vi "FileRichInfo2StringBySecond.vi"(0 "file path (dialog if empty)":path caption="文件路径 （空时为对话框）", 1 "BeginTime(s)":dbl, 2 "EndTime(s)":dbl, 3 "总帧数":i32, 4 "文件类型":string="unknown", 5 "Language":u32) -> (8 "FileInfo":string)   [LabVIEW 2015]
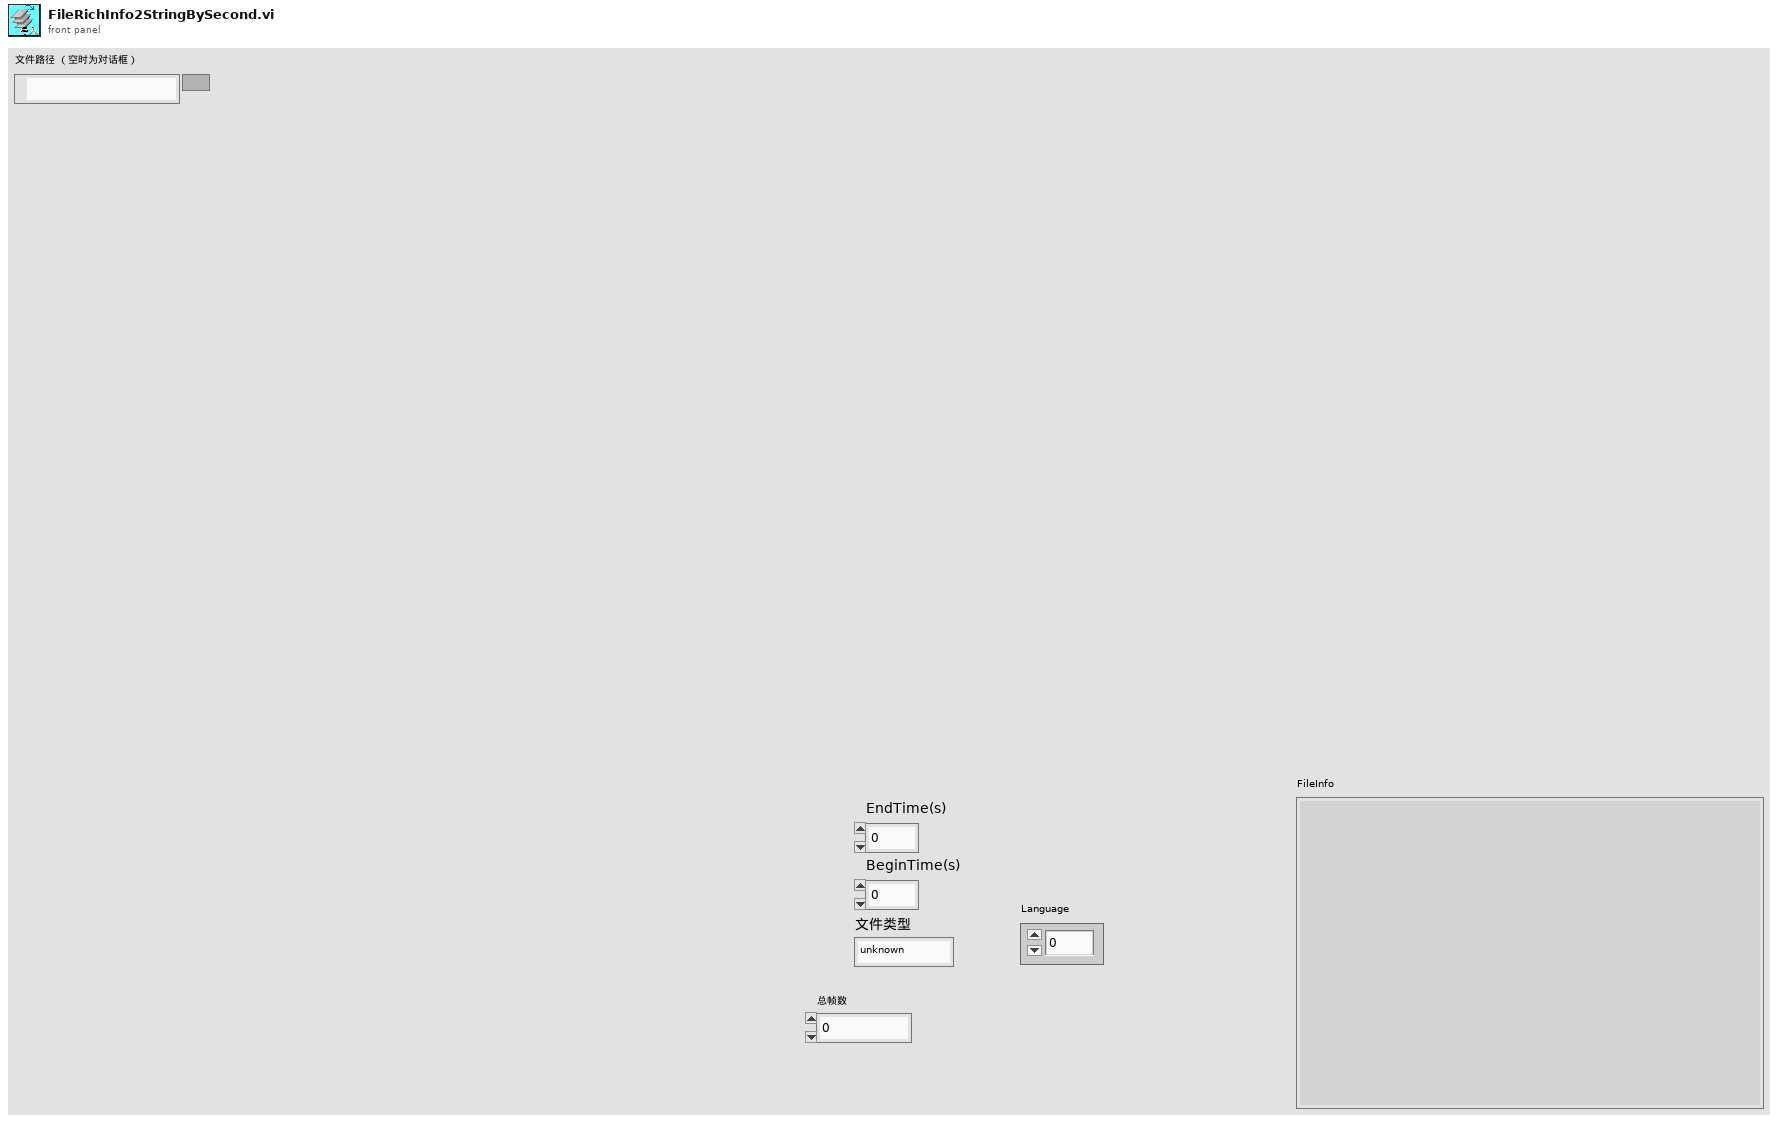
[diagram p1: front panel]
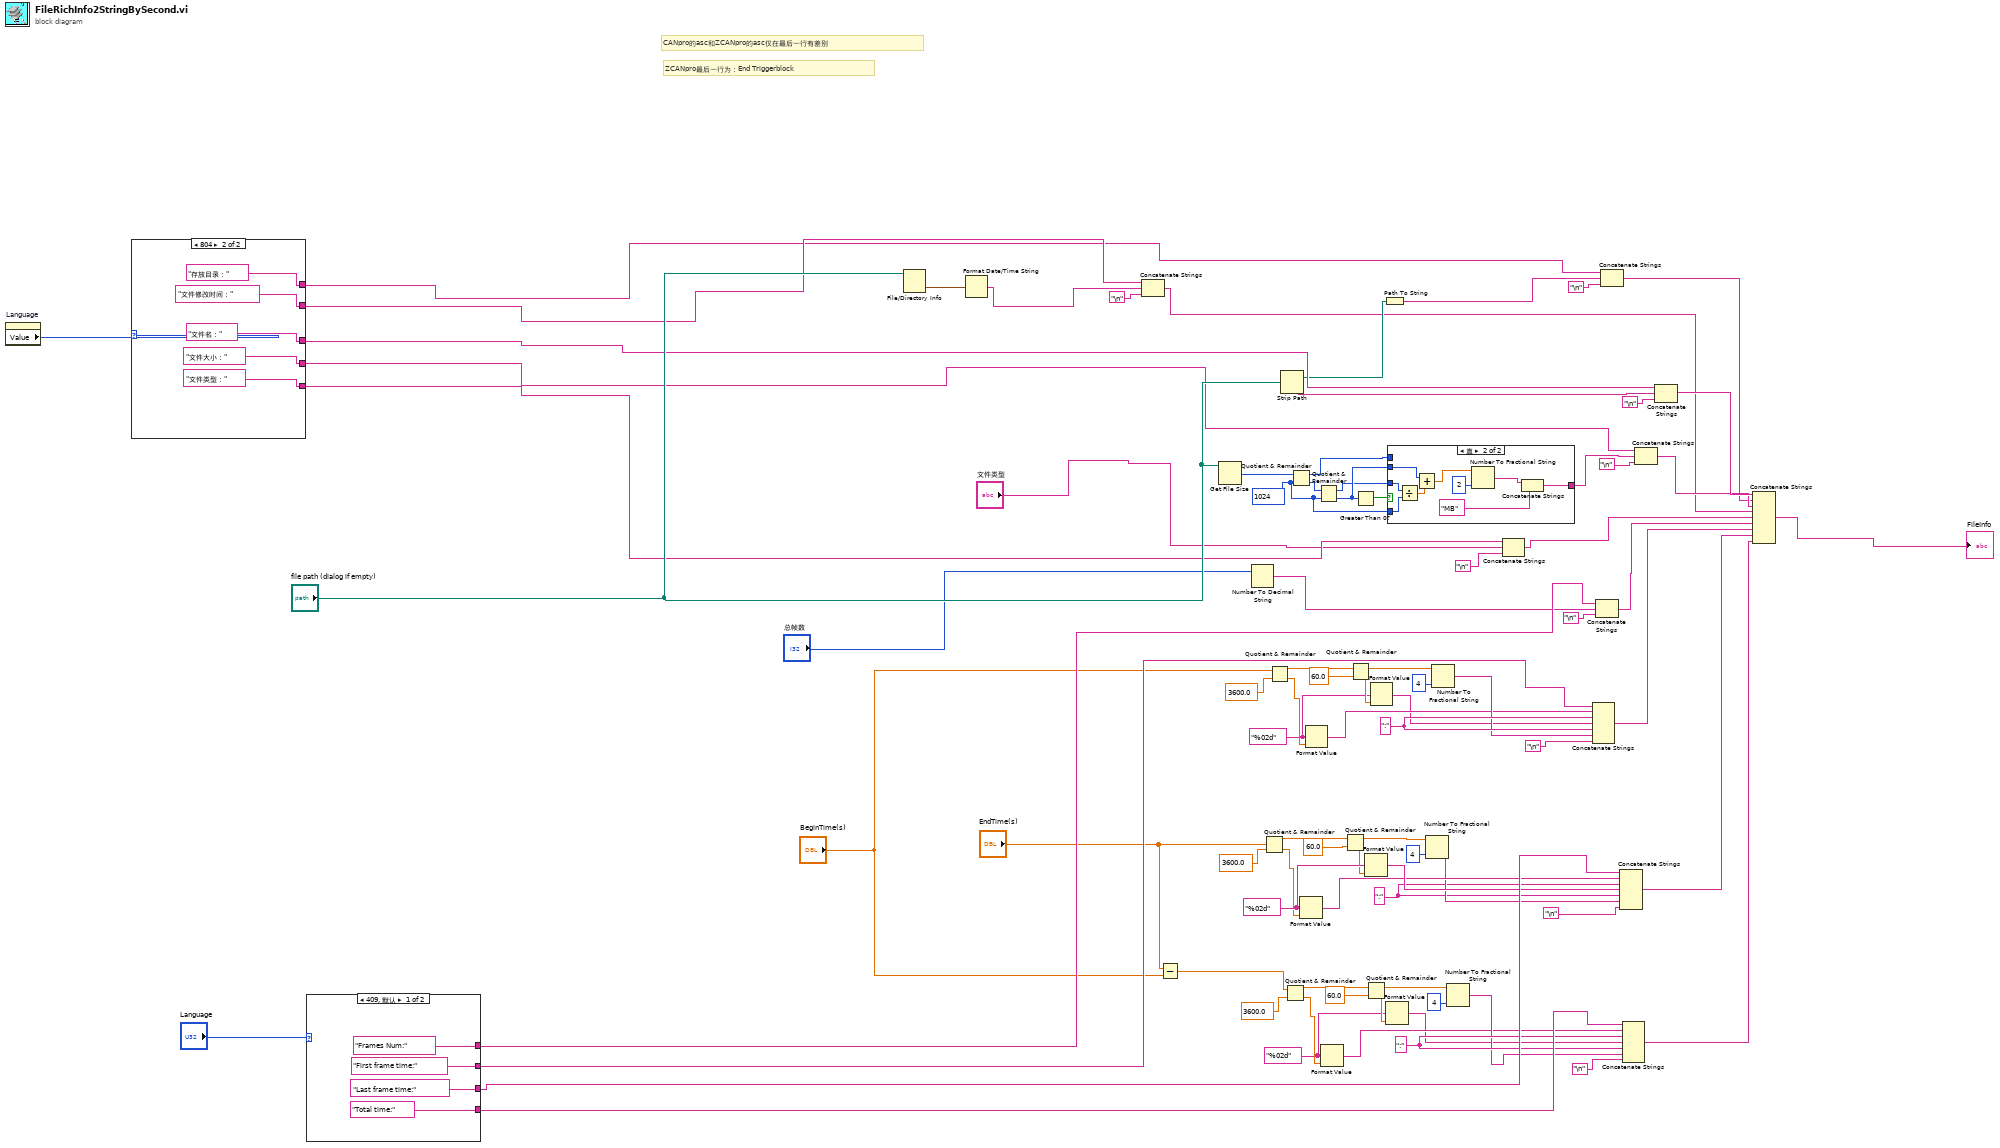
[diagram p0: block diagram]
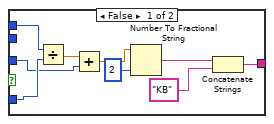
[diagram p2: hidden frame]
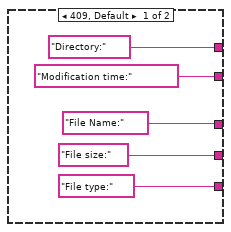
[diagram p3: hidden frame]
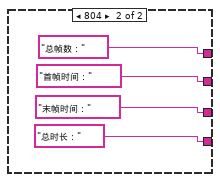
[diagram p4: hidden frame]
diagram:
  w17 = i64 1024 ("y")
  w36 = "%02d" ("格式字符串")
  w42 = ":"
  w60 = "%02d" ("格式字符串")
  w54 = ":"
  w62 = "%02d" ("格式字符串")
  w68 = ":"
  # "ZCANpro最后一行为：End Triggerblock"
  # "CANpro的asc和ZCANpro的asc仅在最后一行有差别"
  n1 = property on="Language" class="DigNum (严格)"() -> ("Value"=w83:u32)  [unwired: 2 in, 2 out]
  n2 = case shown="804" w83 {
    tunnel: ["Modification time:" "文件修改时间："] -> w82
    tunnel: ["Directory:" "存放目录："] -> w79
    tunnel: ["File Name:" "文件名："] -> w80
    tunnel: ["File size:" "文件大小："] -> w78
    tunnel: ["File type:" "文件类型："] -> w81
    frame 409, Default {
    }
    frame 804 {
    }
  }
  n3 = case shown="409, 默认" "Language" {
    tunnel: ["Total time:" "总时长："] -> w77
    tunnel: ["Last frame time:" "末帧时间："] -> w76
    tunnel: ["First frame time:" "首帧时间："] -> w75
    tunnel: ["Frames Num:" "总帧数："] -> w74
    frame 409, Default {
    }
    frame 804 {
    }
  }
  n4 = File/Directory Info(path="file path (dialog if empty)") -> (last mod=w8:timestamp)  [unwired: 1 in, 6 out]
  n5 = Format Date/Time String(seconds (now)=w8) -> (date/time string=w6:string)  [unwired: 2 in]
  n6 = Concatenate Strings(w82, w6, "\n") -> (w5:string)
  n7 = Subtract(x="EndTime(s)", y="BeginTime(s)") -> (x-y=w35:dbl)
  n8 = Get File Size(file="file path (dialog if empty)") -> (size (in bytes)=w20:i64)  [unwired: 1 in, 2 out]
  n9 = Number To Decimal String(number="总帧数") -> (decimal integer string=w23:string)  [unwired: 1 in]
  n10 = Quotient & Remainder(x="EndTime(s)", y=3600.0) -> (x-y*floor(x/y)=w50:dbl, floor(x/y)=w57:dbl)
  n11 = Quotient & Remainder(x="BeginTime(s)", y=3600.0) -> (x-y*floor(x/y)=w72:dbl, floor(x/y)=w65:dbl)
  n12 = Strip Path(path="file path (dialog if empty)") -> (stripped path=w10:path, name=w30:string)
  n13 = Quotient & Remainder(x=w35, y=3600.0) -> (x-y*floor(x/y)=w46:dbl, floor(x/y)=w39:dbl)
  n14 = Quotient & Remainder(x=w20, y=w17) -> (x-y*floor(x/y)=w13:i64, floor(x/y)=w19:i64)
  n15 = Format Value(format string=w60, value (0)=w57) -> (output string=w56:string)  [unwired: 1 in]
  n16 = Format Value(format string=w62, value (0)=w65) -> (output string=w66:string)  [unwired: 1 in]
  n17 = Quotient & Remainder(x=w19, y=w17) -> (x-y*floor(x/y)=w15:i64, floor(x/y)=w16:i64)
  n18 = Format Value(format string=w36, value (0)=w39) -> (output string=w40:string)  [unwired: 1 in]
  n19 = Quotient & Remainder(x=w50, y=60.0) -> (x-y*floor(x/y)=w52:dbl, floor(x/y)=w58:dbl)
  n20 = Quotient & Remainder(x=w72, y=60.0) -> (x-y*floor(x/y)=w70:dbl, floor(x/y)=w64:dbl)
  n21 = Greater Than 0?(x=w16) -> (x > 0?=w18:bool)
  n22 = Format Value(format string=w60, value (0)=w58) -> (output string=w59:string)  [unwired: 1 in]
  n23 = Quotient & Remainder(x=w46, y=60.0) -> (x-y*floor(x/y)=w44:dbl, floor(x/y)=w38:dbl)
  n24 = Format Value(format string=w62, value (0)=w64) -> (output string=w63:string)  [unwired: 1 in]
  n25 = Path To String(path=w10) -> (string=w11:string)
  n26 = Format Value(format string=w36, value (0)=w38) -> (output string=w37:string)  [unwired: 1 in]
  n27 = case shown="真" w18 {
    tunnel: w17 -> [w110 w120]
    tunnel: w16 -> [_ w118]
    tunnel: w15 -> [w108 w121]
    tunnel: [w113 w116] -> w14
    tunnel: w13 -> [w111 _]
    frame False {
      n28 = Divide(x=w111, y=w110) -> (x/y=w109:dbl)
      n29 = Add(x=w109, y=w108) -> (x+y=w107:dbl)
      n30 = Number To Fractional String(number=w107, precision (6)=i16 2 ("精度(6)")) -> (F-format string=w105:string)  [unwired: 2 in]
      n31 = Concatenate Strings(w105, "KB" ("字符串")) -> (w113:string)
    }
    frame True {
      n32 = Divide(x=w121, y=w120) -> (x/y=w119:dbl)
      n33 = Add(x=w118, y=w119) -> (x+y=w117:dbl)
      n34 = Number To Fractional String(number=w117, precision (6)=i16 2 ("精度(6)")) -> (F-format string=w115:string)  [unwired: 2 in]
      n35 = Concatenate Strings(w115, "MB") -> (w116:string)
    }
  }
  n36 = Number To Fractional String(number=w52, precision (6)=i16 4 ("精度(6)")) -> (F-format string=w55:string)  [unwired: 2 in]
  n37 = Number To Fractional String(number=w70, precision (6)=i16 4 ("精度(6)")) -> (F-format string=w67:string)  [unwired: 2 in]
  n38 = Number To Fractional String(number=w44, precision (6)=i16 4 ("精度(6)")) -> (F-format string=w41:string)  [unwired: 2 in]
  n39 = Concatenate Strings(w81, "文件类型", "\n") -> (w27:string)
  n40 = Concatenate Strings(w75, w66, w68, w63, w68, w67, "\n") -> (w61:string)
  n41 = Concatenate Strings(w74, w23, "\n") -> (w24:string)
  n42 = Concatenate Strings(w79, w11, "\n") -> (w9:string)
  n43 = Concatenate Strings(w76, w56, w54, w59, w54, w55, "\n") -> (w48:string)
  n44 = Concatenate Strings(w77, w40, w42, w37, w42, w41, "\n") -> (w34:string)
  n45 = Concatenate Strings(w78, w14, "\n") -> (w21:string)
  n46 = Concatenate Strings(w80, w30, "\n") -> (w29:string)
  n47 = Concatenate Strings(w29, w9, w21, w5, w27, w24, w61, w48, w34) -> (→"FileInfo":string)
